vi "CPP_Aeroprobe_TimeSeries.vi"() -> (5 "Plug in titles":string[](array[string]), 7 "Plug in values":string[](array[string]))   [LabVIEW 2012]
uses:
  Globals/Meas_global.vi
  <vilib>/Analysis/NI_AALBase.lvlib
panel:
  in  "Correction File Path":path
  in  "Apply Phase Correction?":bool=TRUE
  out "DataArray":dbl[](array[numeric])
  out "Zeroes":dbl[](array[numeric])
  out "Progress":dbl(slide) scale=0.0..8192.0
  in  "Old5HoleProbe?":bool
  # "!! 5-hole 1-5 must be connected to Channels 1-5 !!"
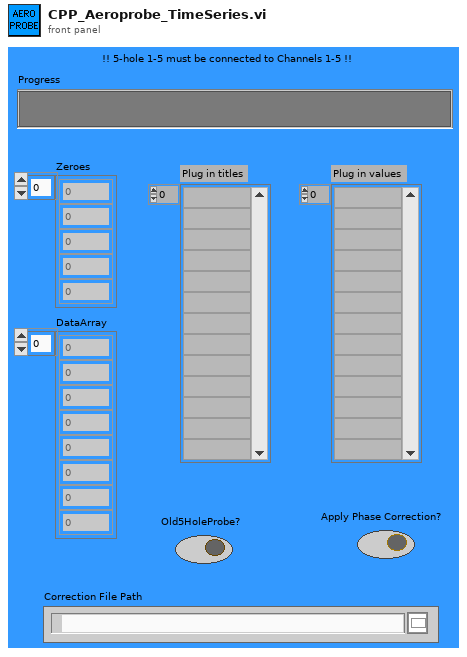
[diagram p1: front panel]
types:
  T1 = typedef "Analysis_info_cluster.ctl" = cluster{"Colour":u32, "Inst type":T2, "Inst name":string, "Symbol":string, "Code name":string, "Extra Info":string, "Inst Array":T3, "Extra Titles":string[], "Extra Values":string[], "U":dbl, "u^2":dbl, "u^3":dbl, "u^4":dbl, "Skew_u":dbl, "Kurt_u":dbl, "Sd Error in Mean":dbl, "% u'/U":dbl, "X":dbl, "Y":dbl, "Z":dbl, "Timescale integral to 25%":dbl, "Sd Error in Variance":dbl, "Calib File":path, "Calib Constants":dbl[], "Output Position":bool, "Full Stats":bool, "Av Sampling Rate":dbl, "Av No of Samples":dbl, "Total Meas Time (s)":dbl, "ADAM Ch Name":string}
  T2 = typedef "Inst_type.ctl" = enum16{"Propeller anemometer", "Raw voltage", "Pressure Transducer", "Pitot-static tube", "Preston tube", "Hot wire", "Cross wire 1", "Cross wire 2", "Generic Linear", "Generic Polynomial", "Generic BackPoly", "Fast FID", "Thermocouple", "Cold wire", "Pulsed Wire", "LDA Vel", "LDA Tran time", "LDA Arr time"}
  T3 = typedef "Instrument_Array.ctl" = enum16{"PWA", "LDA", "Analogue"}
  T4 = cluster{"Analysis Info cluster[0]":T1, "Analysis Info cluster[1]":T1, "Analysis Info cluster[2]":T1, "Analysis Info cluster[3]":T1, "Analysis Info cluster[4]":T1, "Analysis Info cluster[5]":T1, "Analysis Info cluster[6]":T1}
  T5 = typedef "Time_Trace_Cluster.ctl" = cluster{"Weighting":dbl[], "Time (s)":dbl[], "Voltage":dbl[], "Eng Values":dbl[]}
  T6 = cluster{"[0]":dbl, "[1]":dbl, "[2]":dbl, "[3]":dbl, "[4]":dbl}
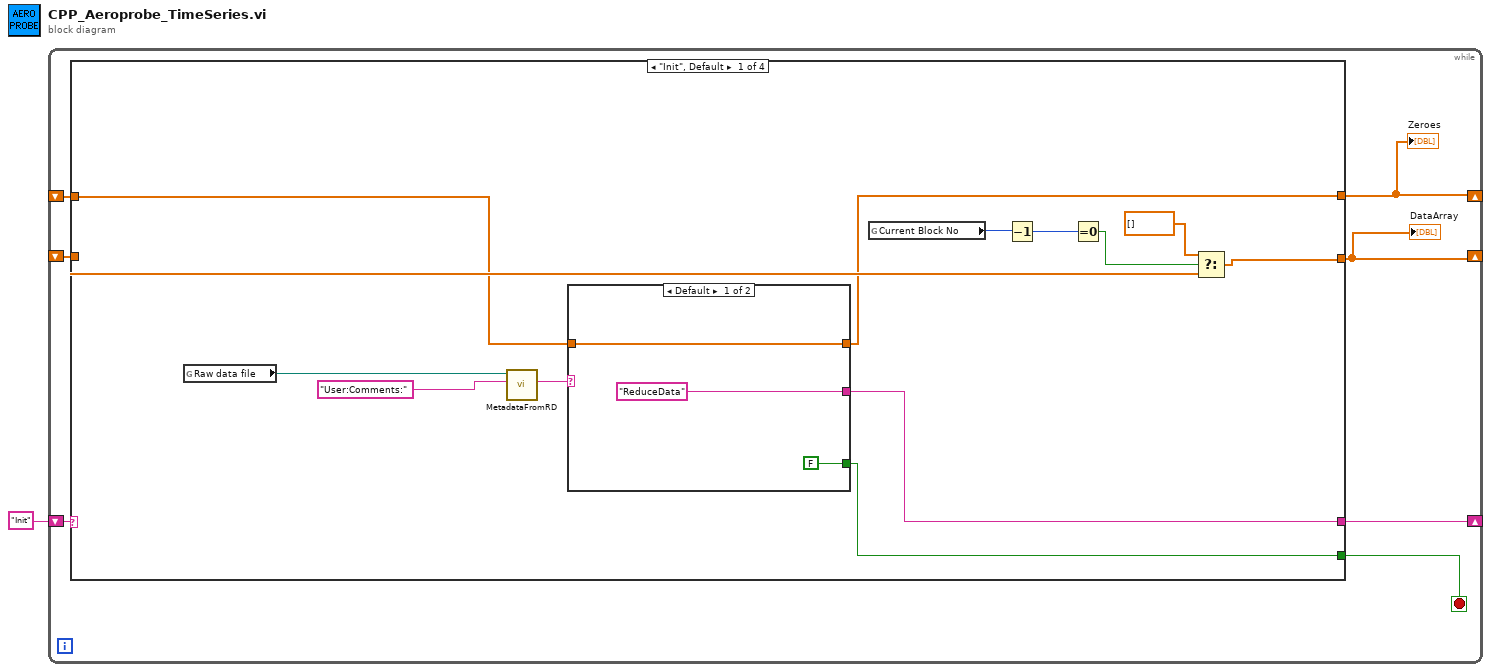
[diagram p0: block diagram]
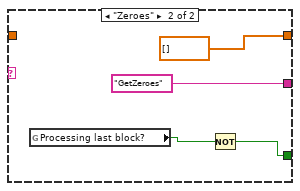
[diagram p2: hidden frame]
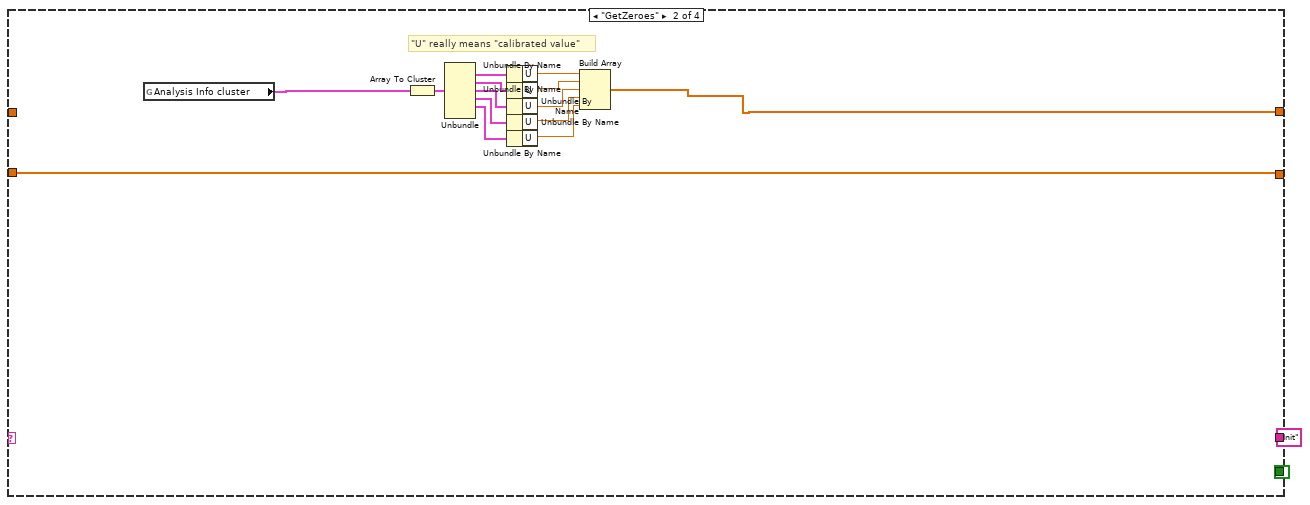
[diagram p3: hidden frame]
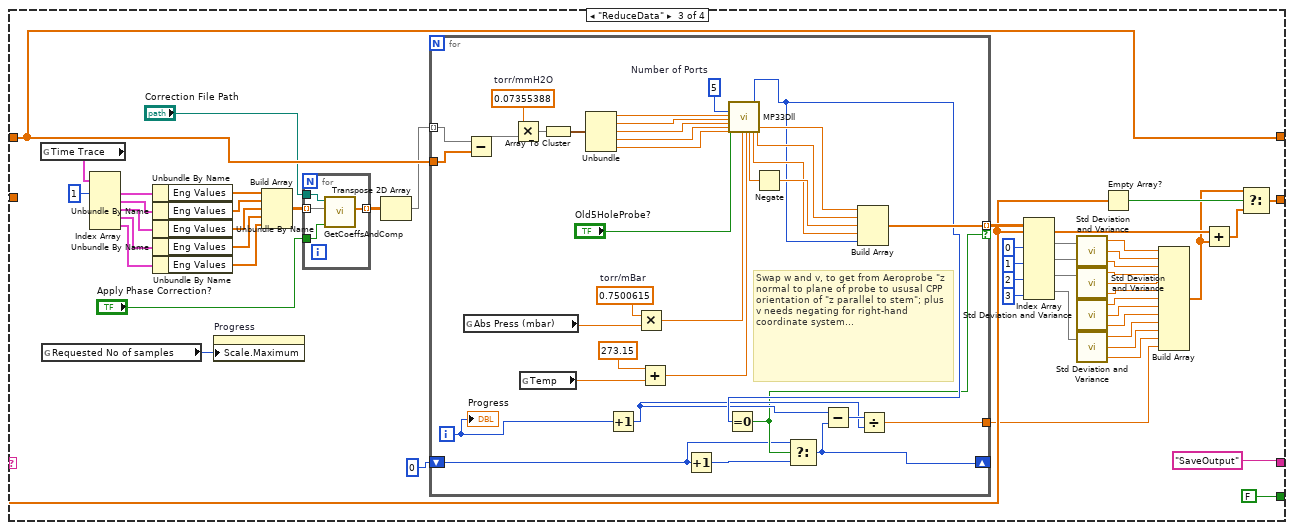
[diagram p4: hidden frame]
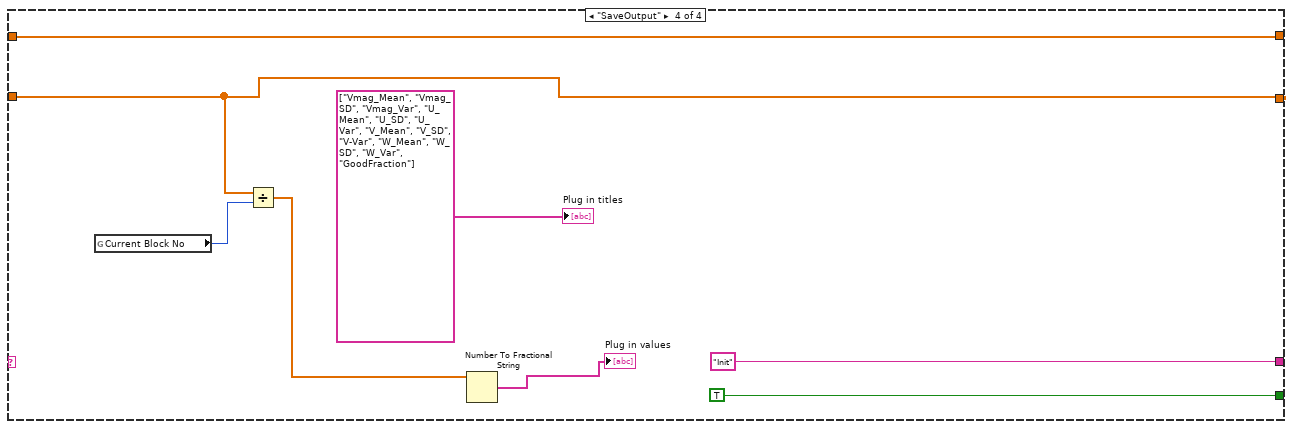
[diagram p5: hidden frame]
diagram:
  n1 = while {
    shift-right: [w7] -> _
    shift-left: "Init" -> [w8]
    shift-right: [w6] -> _
    shift-left: _ -> [w5]
    shift-right: [w4] -> _
    shift-left: _ -> [w3]
    stop <- w2 stop-if-true
    n2 = case shown="\"Init\", Default" w8 {
      tunnel: [w21 "Init" "SaveOutput" "Init"] -> w7
      tunnel: [w11 w31 w92 w139] -> w6
      tunnel: w5 -> [w12 _ w92 w139]
      tunnel: [w14 w29 w55 w133] -> w4
      tunnel: w3 -> [w15 w29 w58 w133]
      tunnel: [w17 TRUE FALSE TRUE] -> w2
      frame "Init", Default {
        n3 = global read "Meas_global.vi" "Raw data file"() -> (w20:path)
        n4 = call "MetadataFromRD.vi"("ChannelName"="User:Comments:", "Raw data file"=w20) -> ("ValueString"=w18:string)  [unwired: 8 in, 1 out]
        n5 = case shown="Default" w18 {
          tunnel: ["ReduceData" "GetZeroes"] -> w21
          tunnel: [FALSE w27] -> w17
          tunnel: w12 -> [w22 _]
          tunnel: [w22 dbl[] [] ("t")] -> w11
          frame Default {
          }
          frame "Zeroes" {
            n6 = global read "Meas_global.vi" "Processing last block?"() -> (w26:bool)
            n7 = Not(x=w26) -> (.not. x?=w27:bool)
          }
        }
        n8 = global read "Meas_global.vi" "Current Block No"() -> (w10:i32)
        n9 = Decrement(x=w10) -> (x-1=w9:i32)
        n10 = Equal To 0?(x=w9) -> (x = 0?=w16:bool)
        n11 = Select(t=dbl[] [], s=w16, f=w15) -> (s? t:f=w14:dbl[])
      }
      frame "GetZeroes" {
        # "\"U\" really means \"calibrated value\""
        n12 = global read "Meas_global.vi" "Analysis Info cluster"() -> (w33:T1[])
        n13 = Array To Cluster(array=w33) -> (cluster=w39:T4)
        n14 = Unbundle(w39) -> ("Analysis Info cluster[1]"=w40:T1, "Analysis Info cluster[2]"=w41:T1, "Analysis Info cluster[3]"=w42:T1, "Analysis Info cluster[4]"=w43:T1, "Analysis Info cluster[5]"=w44:T1)  [unwired: 2 out]
        n15 = Unbundle By Name(w40) -> ("U"=w38:dbl)
        n16 = Unbundle By Name(w41) -> ("U"=w37:dbl)
        n17 = Unbundle By Name(w42) -> ("U"=w36:dbl)
        n18 = Unbundle By Name(w43) -> ("U"=w35:dbl)
        n19 = Unbundle By Name(w44) -> ("U"=w34:dbl)
        n20 = Build Array(w38, w37, w36, w35, w34) -> (w31:dbl[])
      }
      frame "ReduceData" {
        n21 = global read "Meas_global.vi" "Time Trace"() -> (w69:T5[])
        n22 = global read "Meas_global.vi" "Requested No of samples"() -> (w66:i32)
        n23 = Index Array(array=w69, index #1=1 ("index")) -> (element #1=w68:T5, element #2=w78:T5, element #3=w77:T5, element #4=w76:T5, element #5=w75:T5)  [unwired: 4 in]
        n24 = Unbundle By Name(w68) -> ("Eng Values"=w67:dbl[])
        n25 = Unbundle By Name(w78) -> ("Eng Values"=w74:dbl[])
        n26 = Unbundle By Name(w77) -> ("Eng Values"=w73:dbl[])
        n27 = Unbundle By Name(w76) -> ("Eng Values"=w72:dbl[])
        n28 = Unbundle By Name(w75) -> ("Eng Values"=w71:dbl[])
        n29 = property on="Progress" class="Slide (strict)"("Scale.Maximum"=w66) -> ()  [unwired: 2 in, 2 out]
        n30 = Build Array(w67, w74, w73, w72, w71) -> (w48:dbl[][])
        n31 = for {
          tunnel: w48 -> [w97] mode=indexing
          tunnel: [w96] -> w47 mode=indexing
          tunnel: "Apply Phase Correction?" -> [w95]
          tunnel: "Correction File Path" -> [w94]
          n32 = call "GetCoeffsAndComp.vi"("Apply Phase Correction?"=w95, "mutedData"=w97, "TubingCorrectionFile (pre-set!)"=w94) -> ("boostedData"=w96:dbl[])  [unwired: 8 in]
        }
        n33 = Transpose 2D Array(2D array=w47) -> (transposed array=w70:dbl[][])
        n34 = for {
          tunnel: w70 -> [w110] mode=indexing
          tunnel: w92 -> [w109]
          tunnel: [w108] -> w65 mode=indexing if=w100
          shift-right: [w104] -> _
          shift-left: 0 -> [w98]
          tunnel: [w101] -> w50
          i -> [w106]
          w126 = 0.07355388  # torr/mmH2O
          w130 = 0.7500615  # torr/mBar
          w127 = 5  # Number of Ports
          # "Swap w and v, to get from Aeroprobe \"z normal to plane of probe to ususal CPP orientation of \"z parallel to stem\"; plus v needs negating for right-hand coordinate system..."
          n35 = global read "Meas_global.vi" "Abs Press (mbar)"() -> (w112:dbl)
          n36 = Subtract(x=w110, y=w109) -> (x-y=w107:dbl[])
          n37 = Multiply(x=w126, y=w107) -> (x*y=w125:dbl[])
          n38 = global read "Meas_global.vi" "Temp"() -> (w113:dbl)
          n39 = Array To Cluster(array=w125) -> (cluster=w124:T6)
          n40 = Unbundle(w124) -> ("[0]"=w123:dbl, "[1]"=w122:dbl, "[2]"=w121:dbl, "[3]"=w120:dbl, "[4]"=w119:dbl)
          n41 = Increment(x=w106) -> (x+1=w102:i32)
          n42 = Multiply(x=w130, y=w112) -> (x*y=w129:dbl)
          n43 = Add(x=273.15, y=w113) -> (x+y=w131:dbl)
          n44 = Increment(x=w98) -> (x+1=w99:i32)
          n45 = call "MP33Dll.vi"("Old5HoleProbe?"="Old5HoleProbe?", "Number of Ports"=w127, "P1 Torr"=w123, "P2 Torr"=w122, "P3 Torr"=w121, "P4 Torr"=w120, "P5 Torr"=w119, "Pref Torr"=w129, "TTot Kelvin"=w131) -> ("w m/s"=w116:dbl, "return type"=w105:i32, "v m/s"=w114:dbl, "VMagn m/s"=w118:dbl, "u  m/s"=w117:dbl)  [unwired: 8 in, 6 out]
          n46 = Equal To 0?(x=w105) -> (x = 0?=w100:bool)
          n47 = Negate(x=w116) -> (-x=w115:dbl)
          n48 = Select(t=w98, s=w100, f=w99) -> (s? t:f=w104:i32)
          n49 = Subtract(x=w102, y=w104) -> (x-y=w103:i32)
          n50 = Build Array(w118, w117, w115, w114, w105) -> (w108:dbl[])
          n51 = Divide(x=w103, y=w102) -> (x/y=w101:dbl)
          "Progress" <- w106
        }
        n52 = Index Array(array=w65, index (col) #1=0 ("disabled index (col)"), index (col) #2=1 ("index (col)"), index (col) #3=2 ("index (col)"), index (col) #4=3 ("index (col)")) -> (element #1=w91:dbl[], element #2=w90:dbl[], element #3=w89:dbl[], element #4=w88:dbl[])  [unwired: 4 in]
        n53 = call <vilib>:"Std Deviation and Variance.vi"("X"=w91) -> ("mean"=w87:dbl, "standard deviation"=w86:dbl, "variance"=w54:dbl)  [unwired: 1 in]
        n54 = call <vilib>:"Std Deviation and Variance.vi"("X"=w90) -> ("mean"=w85:dbl, "standard deviation"=w83:dbl, "variance"=w53:dbl)  [unwired: 1 in]
        n55 = call <vilib>:"Std Deviation and Variance.vi"("X"=w89) -> ("mean"=w84:dbl, "standard deviation"=w82:dbl, "variance"=w52:dbl)  [unwired: 1 in]
        n56 = call <vilib>:"Std Deviation and Variance.vi"("X"=w88) -> ("mean"=w81:dbl, "standard deviation"=w80:dbl, "variance"=w51:dbl)  [unwired: 1 in]
        n57 = Empty Array?(array=w58) -> (empty?=w57:bool)
        n58 = Build Array(w87, w86, w54, w85, w83, w53, w84, w82, w52, w81, w80, w51, w50) -> (w49:dbl[])
        n59 = Add(x=w58, y=w49) -> (x+y=w56:dbl[])
        n60 = Select(t=w49, s=w57, f=w56) -> (s? t:f=w55:dbl[])
      }
      frame "SaveOutput" {
        n61 = global read "Meas_global.vi" "Current Block No"() -> (w134:i32)
        n62 = Divide(x=w133, y=w134) -> (x/y=w132:dbl[])
        n63 = Number To Fractional String(number=w132) -> (F-format string=→"Plug in values":string[])  [unwired: 3 in]
        "Plug in titles" <- string[] ["Vmag_Mean", "Vmag_SD", "Vmag_Var", "U_Mean", "U_SD", "U_Var", "V_Mean", "V_SD", "V-Var", "W_Mean", "W_SD", "W_Var", "GoodFraction"] ("Plug in titles")
      }
    }
    "Zeroes" <- w6
    "DataArray" <- w4
  }
